vi "Command_Turn_To_Target.vi"(0 "Startup":bool, 1 "Allowable_Error":dbl=3.0, 3 "Timeout":dbl=3.0) -> (5 "Reinit":bool, 6 "Completed":bool=TRUE, 7 "Speeds":dbl[](array[numeric]))   [LabVIEW 2018]
uses:
  Global_Variables/Sensor_Values.vi
panel:
  in  "Kd":dbl=0.02 format="%#_13g"
  in  "Ki":dbl format="%#_13g"
  in  "Kp":dbl=0.1 format="%#_13g"
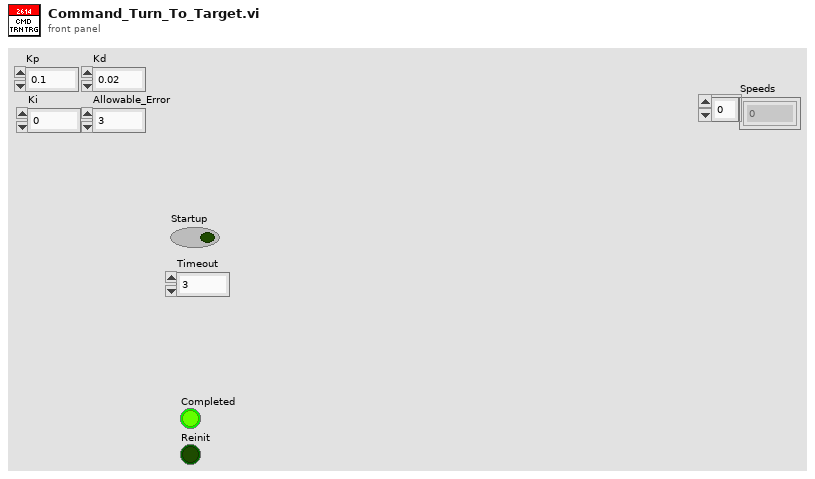
[diagram p1: front panel]
types:
  T1 = cluster{"offsetAngle H":dbl, "offsetAngle V":dbl, "area":dbl, "skew":dbl}
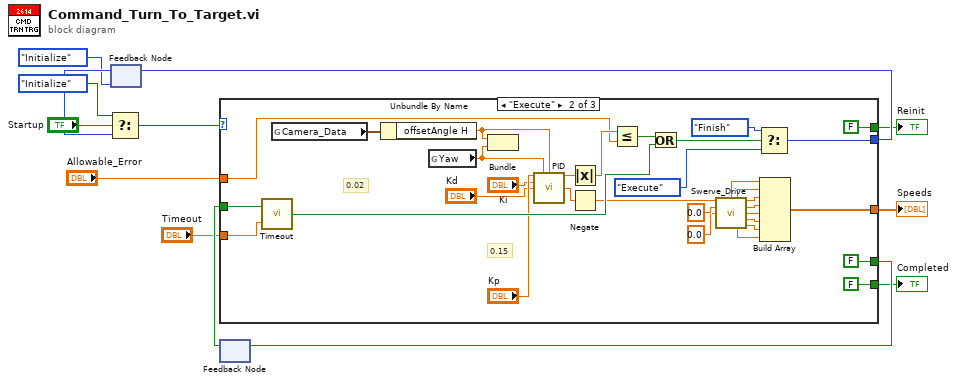
[diagram p0: block diagram]
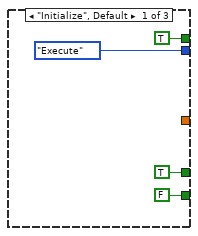
[diagram p2: hidden frame]
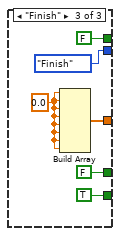
[diagram p3: hidden frame]
diagram:
  n1 = feedback #1(enum16{"Initialize", "Execute", "Finish"}."Initialize" ("f")) -> (w9:enum16{"Initialize", "Execute", "Finish"})
  n2 = Select(t=enum16{"Initialize", "Execute", "Finish"}."Initialize", s="Startup", f=w9) -> (s? t:f=w13:enum16{"Initialize", "Execute", "Finish"})
  n3 = feedback #2() -> (w7:bool)  [unwired: 1 in]
  n4 = case shown="\"Execute\"" w13 {
    tunnel: [enum16{"Initialize", "Execute", "Finish"}."Execute" w47 enum16{"Initialize", "Execute", "Finish"}."Finish" ("f")] -> w10
    tunnel: w7 -> [_ w45 _]
    tunnel: [TRUE FALSE FALSE] -> w8
    tunnel: [FALSE FALSE TRUE] -> w6
    tunnel: [TRUE FALSE FALSE] -> w5
    tunnel: "Timeout" -> [_ w41 _]
    tunnel: [_ w32 w52] -> w2
    tunnel: "Allowable_Error" -> [_ w18 _]
    frame "Initialize", Default {
    }
    frame "Execute" {
      # "0.02"
      # "0.15"
      n5 = call "Timeout.vi"("Timeout"=w41, "Initialize"=w45) -> ("Timed Out?"=w42:bool)
      n6 = global read "Sensor_Values.vi" "Camera_Data"() -> (w20:T1)
      n7 = Unbundle By Name(w20) -> ("offsetAngle H"=w19:dbl)
      n8 = global read "Sensor_Values.vi" "Yaw"() -> (w28:dbl)
      n9 = Bundle("offsetAngle H"=w19, "Yaw"=w28) -> ()  [unwired: 1 in, 1 out]
      n10 = call "PID.vi"("Kp"="Kp", "Process Variable"=w28, "Goal"=w19, "Ki"="Ki", "Kd"="Kd") -> ("Current Error"=w22:dbl, "Command"=w24:dbl)  [unwired: 8 in, 1 out]
      n11 = Absolute Value(x=w22) -> (abs(x)=w21:dbl)
      n12 = Negate(x=w24) -> (-x=w23:dbl)
      n13 = Less Or Equal?(x=w21, y=w18) -> (x <= y?=w27:bool)
      n14 = Or(x=w27, y=w42) -> (x .or. y?=w43:bool)
      n15 = call "Swerve_Drive.vi"("Z"=w23, "Y"=0.0, "X"=0.0) -> ("Back Left Spin Speed"=w40:dbl, "Back Right Spin Speed"=w39:dbl, "Front Left Spin Speed"=w38:dbl, "Front Right Spin Speed"=w37:dbl, "Back Left Motor Power"=w36:dbl, "Back Right Motor Power"=w35:dbl, "Front Right Motor Power"=w33:dbl, "Front Left Motor Power"=w34:dbl)  [unwired: 5 in]
      n16 = Select(t=enum16{"Initialize", "Execute", "Finish"}."Finish", s=w43, f=enum16{"Initialize", "Execute", "Finish"}."Execute") -> (s? t:f=w47:enum16{"Initialize", "Execute", "Finish"})
      n17 = Build Array(w40, w39, w38, w37, w36, w35, w34, w33) -> (w32:dbl[])
    }
    frame "Finish" {
      w51 = 0.0 ("element")
      n18 = Build Array(w51, w51, w51, w51, w51, w51, w51, w51) -> (w52:dbl[])
    }
  }
  "Completed" <- w6
  "Reinit" <- w5
  "Speeds" <- w2
  n19 = feedback-in #1(w10) -> ()
  n20 = feedback-in #2(w8) -> ()
